vi "Initialize 8 NEO Swerve Drive.vi"() -> (0 "error out":errorcluster, 3 "Motors":T1={"Drive Motors (NEO)"={"Left Front"={"DeviceStatus"={"status"=FALSE, "code"=0, "source"=""}, "Type"=enum."PWM", "PWM"={"PWM Channel"=enum."Invalid", "DeadBand"={"Name"="", "maxPositivePwm"=0, "minPositivePwm"=0, "centerPwm"=0, "maxNegativePwm"=0, "minNegativePwm"=0, "angularRange"=0}}, "CAN"={"Device Number"=0, "SetOutput VI Ref"=variant, "GetOutput VI Ref"=variant, "Enable VI Ref"=variant, "Disable VI Ref"=variant, "Data"=variant}, "Invert"=FALSE, "DIO PWM"={"PWM \"Enable\" Channel"=enum."Invalid", "DIOChannel"=enum."Invalid", "PWM Rate"=0.0}}, "Left Back"={"DeviceStatus"={"status"=FALSE, "code"=0, "source"=""}, "Type"=enum."PWM", "PWM"={"PWM Channel"=enum."Invalid", "DeadBand"={"Name"="", "maxPositivePwm"=0, "minPositivePwm"=0, "centerPwm"=0, "maxNegativePwm"=0, "minNegativePwm"=0, "angularRange"=0}}, "CAN"={"Device Number"=0, "SetOutput VI Ref"=variant, "GetOutput VI Ref"=variant, "Enable VI Ref"=variant, "Disable VI Ref"=variant, "Data"=variant}, "Invert"=FALSE, "DIO PWM"={"PWM \"Enable\" Channel"=enum."Invalid", "DIOChannel"=enum."Invalid", "PWM Rate"=0.0}}, "Right Front"={"DeviceStatus"={"status"=FALSE, "code"=0, "source"=""}, "Type"=enum."PWM", "PWM"={"PWM Channel"=enum."Invalid", "DeadBand"={"Name"="", "maxPositivePwm"=0, "minPositivePwm"=0, "centerPwm"=0, "maxNegativePwm"=0, "minNegativePwm"=0, "angularRange"=0}}, "CAN"={"Device Number"=0, "SetOutput VI Ref"=variant, "GetOutput VI Ref"=variant, "Enable VI Ref"=variant, "Disable VI Ref"=variant, "Data"=variant}, "Invert"=FALSE, "DIO PWM"={"PWM \"Enable\" Channel"=enum."Invalid", "DIOChannel"=enum."Invalid", "PWM Rate"=0.0}}, "Right Back"={"DeviceStatus"={"status"=FALSE, "code"=0, "source"=""}, "Type"=enum."PWM", "PWM"={"PWM Channel"=enum."Invalid", "DeadBand"={"Name"="", "maxPositivePwm"=0, "minPositivePwm"=0, "centerPwm"=0, "maxNegativePwm"=0, "minNegativePwm"=0, "angularRange"=0}}, "CAN"={"Device Number"=0, "SetOutput VI Ref"=variant, "GetOutput VI Ref"=variant, "Enable VI Ref"=variant, "Disable VI Ref"=variant, "Data"=variant}, "Invert"=FALSE, "DIO PWM"={"PWM \"Enable\" Channel"=enum."Invalid", "DIOChannel"=enum."Invalid", "PWM Rate"=0.0}}}, "Steer Motors (NEO)"={"Left Front"={"DeviceStatus"={"status"=FALSE, "code"=0, "source"=""}, "Type"=enum."PWM", "PWM"={"PWM Channel"=enum."Invalid", "DeadBand"={"Name"="", "maxPositivePwm"=0, "minPositivePwm"=0, "centerPwm"=0, "maxNegativePwm"=0, "minNegativePwm"=0, "angularRange"=0}}, "CAN"={"Device Number"=0, "SetOutput VI Ref"=variant, "GetOutput VI Ref"=variant, "Enable VI Ref"=variant, "Disable VI Ref"=variant, "Data"=variant}, "Invert"=FALSE, "DIO PWM"={"PWM \"Enable\" Channel"=enum."Invalid", "DIOChannel"=enum."Invalid", "PWM Rate"=0.0}}, "Left Back"={"DeviceStatus"={"status"=FALSE, "code"=0, "source"=""}, "Type"=enum."PWM", "PWM"={"PWM Channel"=enum."Invalid", "DeadBand"={"Name"="", "maxPositivePwm"=0, "minPositivePwm"=0, "centerPwm"=0, "maxNegativePwm"=0, "minNegativePwm"=0, "angularRange"=0}}, "CAN"={"Device Number"=0, "SetOutput VI Ref"=variant, "GetOutput VI Ref"=variant, "Enable VI Ref"=variant, "Disable VI Ref"=variant, "Data"=variant}, "Invert"=FALSE, "DIO PWM"={"PWM \"Enable\" Channel"=enum."Invalid", "DIOChannel"=enum."Invalid", "PWM Rate"=0.0}}, "Right Front"={"DeviceStatus"={"status"=FALSE, "code"=0, "source"=""}, "Type"=enum."PWM", "PWM"={"PWM Channel"=enum."Invalid", "DeadBand"={"Name"="", "maxPositivePwm"=0, "minPositivePwm"=0, "centerPwm"=0, "maxNegativePwm"=0, "minNegativePwm"=0, "angularRange"=0}}, "CAN"={"Device Number"=0, "SetOutput VI Ref"=variant, "GetOutput VI Ref"=variant, "Enable VI Ref"=variant, "Disable VI Ref"=variant, "Data"=variant}, "Invert"=FALSE, "DIO PWM"={"PWM \"Enable\" Channel"=enum."Invalid", "DIOChannel"=enum."Invalid", "PWM Rate"=0.0}}, "Right Back"={"DeviceStatus"={"status"=FALSE, "code"=0, "source"=""}, "Type"=enum."PWM", "PWM"={"PWM Channel"=enum."Invalid", "DeadBand"={"Name"="", "maxPositivePwm"=0, "minPositivePwm"=0, "centerPwm"=0, "maxNegativePwm"=0, "minNegativePwm"=0, "angularRange"=0}}, "CAN"={"Device Number"=0, "SetOutput VI Ref"=variant, "GetOutput VI Ref"=variant, "Enable VI Ref"=variant, "Disable VI Ref"=variant, "Data"=variant}, "Invert"=FALSE, "DIO PWM"={"PWM \"Enable\" Channel"=enum."Invalid", "DIOChannel"=enum."Invalid", "PWM Rate"=0.0}}}, "PigeonIMUDevRef"={"DeviceStatus"={"status"=FALSE, "code"=0, "source"=""}, "Device Number"=0, "Type"=352321536, "Device ID"=0, "Handle"=0, "UsageFrame"=0, "Library Path"=path ""}, "Radii (ft)"={"Left Front Position"=[], "Left Back Position"=[], "Right Front Position"=[], "Right Back Position"=[]}} {"PigeonIMUDevRef"."Type" items=["CAN"=352321536, "TalonSRX"=33554432]; "Radii (ft)"."Right Back Position" format="%.2f"; "Radii (ft)"."Right Front Position" format="%.2f"; "Radii (ft)"."Left Back Position" format="%.2f"; "Radii (ft)"."Left Front Position" format="%.2f"})   [LabVIEW 2025]
doc: "Creates a cluster of 4 motors (order is left-front, left-back, right-front, right-back) initialized with PID coefficients and status frame reduction"
uses:
  Type Definitions/Hardware/Swerve Drives/(NEO-NEO-ThroughBore-Pigeon2) Swerve.ctl
  Type Definitions/Hardware/4 Motor Sets/(NEO & NEO 550) 4 Motor Set.ctl
  <vilib>/Rock Robotics/WPI/MotorControl/WPI_MotorControlDeviceRef.ctl
  <vilib>/Rock Robotics/WPI/MotorControl/WPI_MotorControlType.ctl
  <vilib>/Rock Robotics/SystemInterfaces/DIO/FPGA_DIOPWMChannel.ctl
  <vilib>/Rock Robotics/WPI/PWM/WPI_PWMDeadband.ctl
  <vilib>/Rock Robotics/SystemInterfaces/DIO/FPGA_DIOChannel.ctl
  <vilib>/Rock Robotics/WPI/ThirdParty/Phoenix-LabVIEW/Pigeon IMU/CTRE_PigeonIMU_DeviceRef.ctl
  <vilib>/Rock Robotics/WPI/ThirdParty/Phoenix-LabVIEW/Pigeon IMU/CTRE_PigeonIMU_ConnectionType.ctl
  Type Definitions/Data/Pod Positions.ctl
  Type Definitions/Hardware/Swerve Configs/NEO-NEO-ThroughBore-Pigeon2 Swerve Config.ctl
  <vilib>/Rock Robotics/WPI/ThirdParty/REV Robotics/REVLib/Typedef/SPARK Feed Forward Gains.ctl
  <vilib>/Rock Robotics/WPI/ThirdParty/REV Robotics/REVLib/Typedef/Spark MAX Idle Mode.ctl
  <vilib>/Rock Robotics/WPI/ThirdParty/REV Robotics/REVLib/Typedef/SPARK Feedback Sensor.ctl
  <vilib>/Rock Robotics/WPI/ThirdParty/REV Robotics/REVLib/Typedef/Spark MAX Status Frames.ctl
  <vilib>/Rock Robotics/WPI/ThirdParty/REV Robotics/REVLib/Typedef/Closed Loop Voltage Mode.ctl
  <vilib>/Rock Robotics/WPI/ThirdParty/REV Robotics/REVLib/Typedef/Spark MAX Hall Sensor Average Depth Size.ctl
  <vilib>/Rock Robotics/WPI/ThirdParty/REV Robotics/REVLib/SubVI/Public/SPARK Open Brushless.vi
  <vilib>/Rock Robotics/WPI/ThirdParty/REV Robotics/REVLib/SubVI/Public/SPARK Configure Power Smart Current Limit.vi
  <vilib>/Rock Robotics/WPI/ThirdParty/REV Robotics/REVLib/SubVI/Public/SPARK Configure Closed Loop Basic.vi
  <vilib>/Rock Robotics/WPI/ThirdParty/REV Robotics/REVLib/SubVI/Public/SPARK Configure Encoder Conversion Factors.vi
  <vilib>/Rock Robotics/WPI/ThirdParty/REV Robotics/REVLib/SubVI/Public/SPARK Configure Closed Loop Position Wrapping.vi
  <vilib>/Rock Robotics/WPI/ThirdParty/REV Robotics/REVLib/SubVI/Public/SPARK Configure Basic Idle Mode.vi
  <vilib>/Rock Robotics/WPI/ThirdParty/REV Robotics/REVLib/SubVI/Public/SPARK Configure Closed Loop Voltage Mode.vi
  <vilib>/Rock Robotics/WPI/ThirdParty/REV Robotics/REVLib/SubVI/Public/SPARK Configure Encoder Velocity Filtering UVW.vi
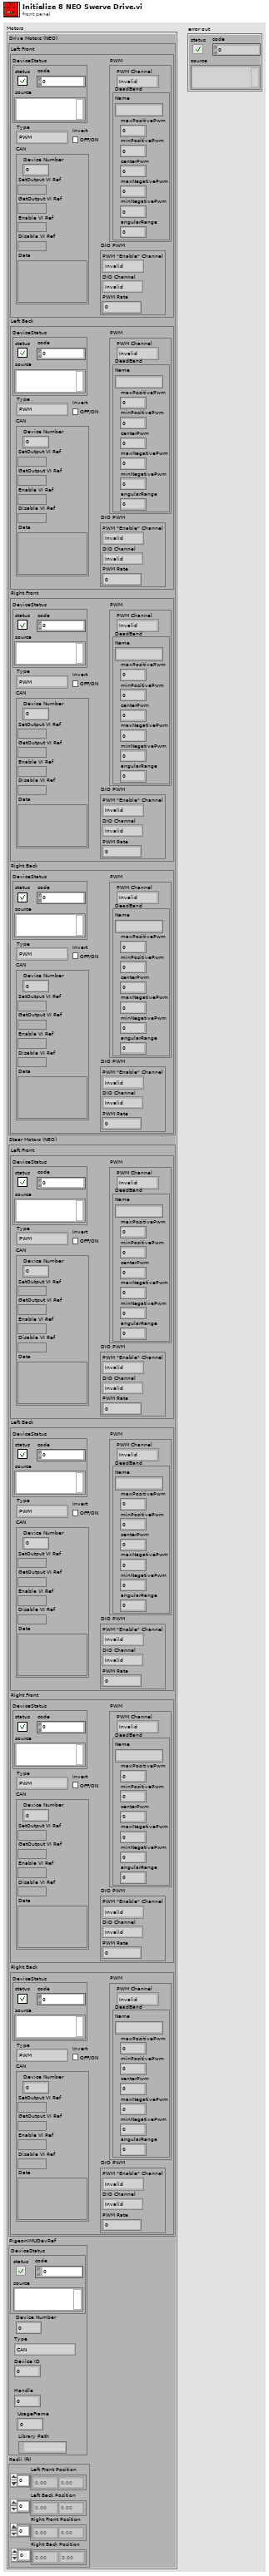
[diagram p1: front panel]
types:
  T1 = typedef "(NEO-NEO-ThroughBore-Pigeon2) Swerve.ctl" = cluster{"Drive Motors (NEO)":T2, "Steer Motors (NEO)":T2, "PigeonIMUDevRef":T8, "Radii (ft)":T10}
  T2 = typedef "(NEO & NEO 550) 4 Motor Set.ctl" = cluster{"Left Front":T3, "Left Back":T3, "Right Front":T3, "Right Back":T3}
  T3 = typedef "WPI_MotorControlDeviceRef.ctl" = cluster{"DeviceStatus":errorcluster, "Type":T4, "PWM":cluster{"PWM Channel":T5, "DeadBand":T6}, "CAN":cluster{"Device Number":u8, "SetOutput VI Ref":variant, "GetOutput VI Ref":variant, "Enable VI Ref":variant, "Disable VI Ref":variant, "Data":variant}, "Invert":bool, "DIO PWM":cluster{"PWM \"Enable\" Channel":T5, "DIOChannel":T7, "PWM Rate":dbl}}
  T4 = typedef "WPI_MotorControlType.ctl" = enum16{"PWM", "CAN", "DIO PWM"}
  T5 = typedef "FPGA_DIOPWMChannel.ctl" = enum8{"PWM 0", "PWM 1", "PWM 2", "PWM 3", "PWM 4", "PWM 5", "PWM 6", "PWM 7", "PWM 8", "PWM 9", "PWM MXP 0", "PWM MXP 1", "PWM MXP 2", "PWM MXP 3", "PWM MXP 4", "PWM MXP 5", "PWM MXP 6", "PWM MXP 7", "PWM MXP 8", "PWM MXP 9", "Invalid"}
  T6 = typedef "WPI_PWMDeadband.ctl" = cluster{"Name":string, "maxPositivePwm":i32, "minPositivePwm":i32, "centerPwm":i32, "maxNegativePwm":i32, "minNegativePwm":i32, "angularRange":u16}
  T7 = typedef "FPGA_DIOChannel.ctl" = enum8{"DIO 0", "DIO 1", "DIO 2", "DIO 3", "DIO 4", "DIO 5", "DIO 6", "DIO 7", "DIO 8", "DIO 9", "DIO MXP 0", "DIO MXP 1", "DIO MXP 2", "DIO MXP 3", "DIO MXP 4", "DIO MXP 5", "DIO MXP 6", "DIO MXP 7", "DIO MXP 8", "DIO MXP 9", "DIO MXP 10", "DIO MXP 11", "DIO MXP 12", "DIO MXP 13", "DIO MXP 14", "DIO MXP 15", "SPI Port CS1", "SPI Port CS2", "SPI Port CS3", "SPI Port MISO", "SPI Port MOSI", "Invalid"}
  T8 = typedef "CTRE_PigeonIMU_DeviceRef.ctl" = cluster{"DeviceStatus":errorcluster, "Device Number":u8, "Type":T9, "Device ID":u32, "Handle":u64, "UsageFrame":u32, "Library Path":path}
  T9 = typedef "CTRE_PigeonIMU_ConnectionType.ctl" = u32
  T10 = typedef "Pod Positions.ctl" = cluster{"Left Front Position":dbl[], "Left Back Position":dbl[], "Right Front Position":dbl[], "Right Back Position":dbl[]}
  T11 = typedef "NEO-NEO-ThroughBore-Pigeon2 Swerve Config.ctl" = cluster{"Drive Motor CAN IDs":cluster{"LF CAN ID":dbl, "LB CAN ID":dbl, "RF CAN ID":dbl, "RB CAN ID":dbl}, "Steer Motor CAN IDs":cluster{"LF CAN ID":dbl, "LB CAN ID":dbl, "RF CAN ID":dbl, "RB CAN ID":dbl}, "Drive PID Gains":cluster{cluster{"P Gain":dbl, "I Gain":dbl, "D Gain":dbl}, "Feed Forward Gains":T12, "I Zone":dbl, "Min Output":dbl, "Max Output":dbl}, "Steer PID Gains":cluster{cluster{"P Gain":dbl, "I Gain":dbl, "D Gain":dbl}, "Feed Forward Gains":T12, "I Zone":dbl, "Min Output":dbl, "Max Output":dbl}, "Pigeon 2 Refnum":string, "Pod Locations (ft)":T10}
  T12 = typedef "SPARK Feed Forward Gains.ctl" = cluster{"kV":dbl, "kS":dbl, "kA":dbl, "kG":dbl, "kCos":dbl, "kCosRatio":dbl}
  T13 = cluster{"LF CAN ID":dbl, "LB CAN ID":dbl, "RF CAN ID":dbl, "RB CAN ID":dbl}
  T14 = cluster{cluster{"P Gain":dbl, "I Gain":dbl, "D Gain":dbl}, "Feed Forward Gains":T12, "I Zone":dbl, "Min Output":dbl, "Max Output":dbl}
  T15 = typedef "Spark MAX Hall Sensor Average Depth Size.ctl" = enum16{"1", "2", "4", "8"}
  T16 = typedef "SPARK Feedback Sensor.ctl" = enum16{"No Sensor", "Primary Encoder", "Analog Sensor", "Alternate or External Encoder", "Duty Cycle Sensor"}
  T17 = typedef "Closed Loop Voltage Mode.ctl" = enum16{"Disabled", "Voltage Output", "Voltage Compensation"}
  T18 = typedef "Spark MAX Status Frames.ctl" = enum16{"Status 0", "Status 1", "Status 2", "Status 3", "Status 4", "Status 5", "Status 6", "Status 7"}
  T19 = typedef "Spark MAX Idle Mode.ctl" = enum16{"Coast", "Brake"}
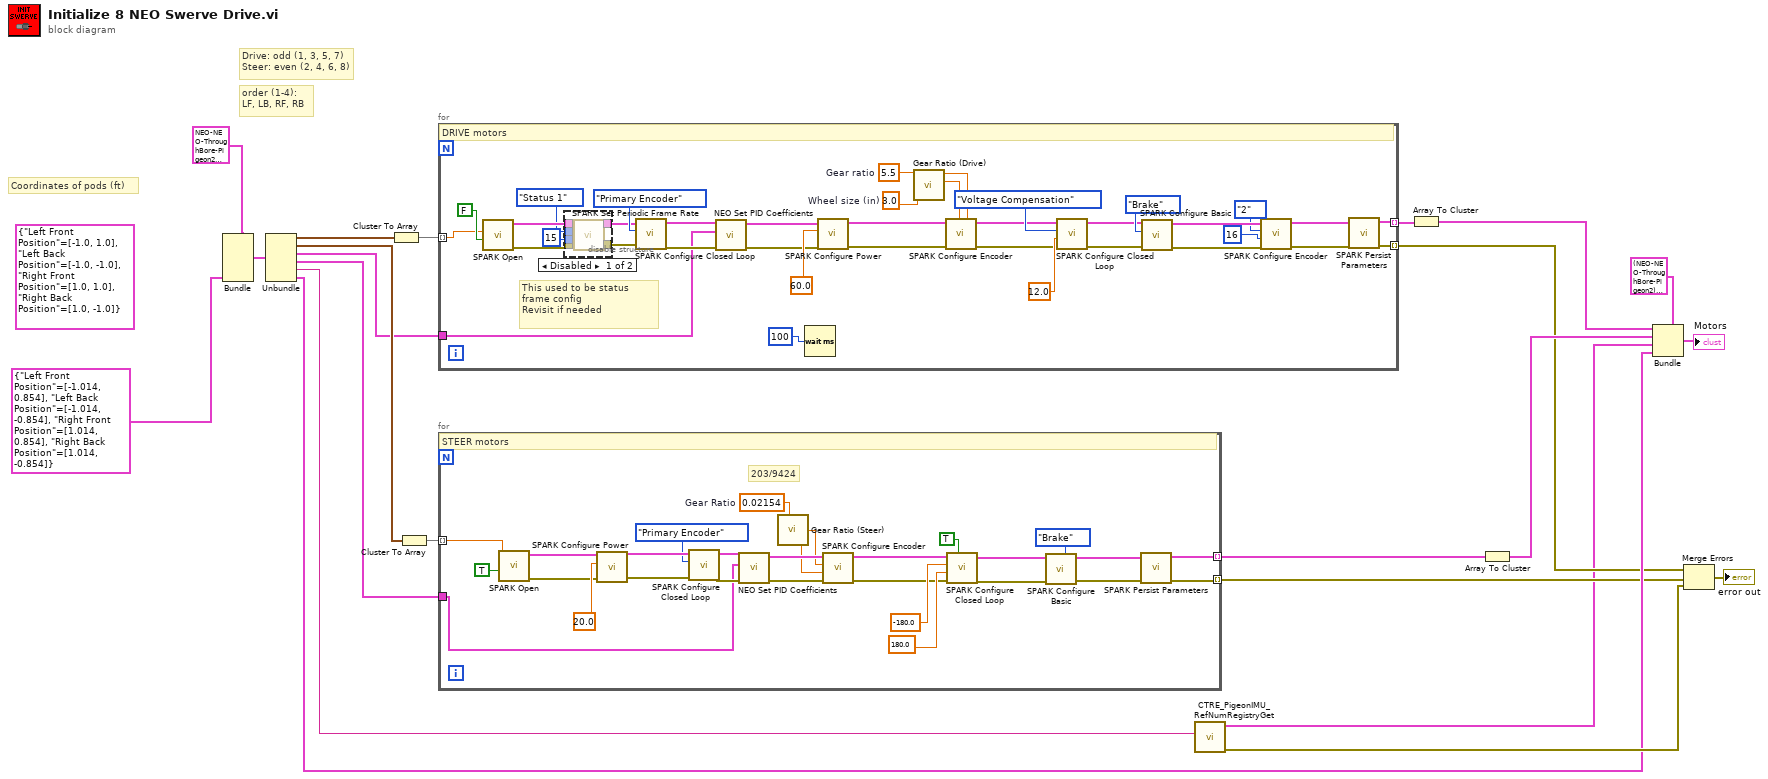
[diagram p0: block diagram]
diagram:
  (unwired) T10 {"Left Front Position"=[-1.0, 1.0], "Left Back Position"=[-1.0, -1.0], "Right Front Position"=[1.0, 1.0], "Right Back Position"=[1.0, -1.0]} ("Radii (ft)")
  # "Drive: odd (1, 3, 5, 7)\nSteer: even (2, 4, 6, 8)"
  # "Coordinates of pods (ft)"
  # "order (1-4):\nLF, LB, RF, RB"
  n1 = Bundle(cluster=T11 {"Drive Motor CAN IDs"={"LF CAN ID"=1.0, "LB CAN ID"=3.0, "RF CAN ID"=5.0, "RB CAN ID"=7.0}, "Steer Motor CAN IDs"={"LF CAN ID"=2.0, "LB CAN ID"=4.0, "RF CAN ID"=6.0, "RB CAN ID"=8.0}, "Drive PID Gains"={{"P Gain"=0.12, "I Gain"=0.0, "D Gain"=0.0}, "Feed Forward Gains"={"kV"=0.08, "kS"=0.0, "kA"=0.0, "kG"=0.0, "kCos"=0.0, "kCosRatio"=0.0}, "I Zone"=0.0, "Min Output"=-1.0, "Max Output"=1.0}, "Steer PID Gains"={{"P Gain"=0.08, "I Gain"=0.0, "D Gain"=0.0}, "Feed Forward Gains"={"kV"=0.0, "kS"=0.0, "kA"=0.0, "kG"=0.0, "kCos"=0.0, "kCosRatio"=0.0}, "I Zone"=0.0, "Min Output"=-1.0, "Max Output"=1.0}, "Pigeon 2 Refnum"="IMU", "Pod Locations (ft)"={"Left Front Position"=[], "Left Back Position"=[], "Right Front Position"=[], "Right Back Position"=[]}} ("Swerve Config"), "Pod Locations (ft)"=T10 {"Left Front Position"=[-1.014, 0.854], "Left Back Position"=[-1.014, -0.854], "Right Front Position"=[1.014, 0.854], "Right Back Position"=[1.014, -0.854]} ("Radii (ft)")) -> (w18:T11)  [unwired: 5 in]
  n2 = Unbundle(w18) -> ("Drive Motor CAN IDs"=w17:T13, "Steer Motor CAN IDs"=w16:T13, "Drive PID Gains"=w13:T14, "Steer PID Gains"=w12:T14, "Pigeon 2 Refnum"=w11:string, "Pod Locations (ft)"=w10:T10)
  n3 = Cluster To Array(cluster=w17) -> (array=w22:dbl[])
  n4 = Cluster To Array(cluster=w16) -> (array=w21:dbl[])
  n5 = for {
    tunnel: w22 -> [w33] mode=indexing
    tunnel: w13 -> [w27]
    tunnel: [w24] -> w8 mode=indexing
    tunnel: [w23] -> w4 mode=indexing
    w53 = 3.0  # Wheel size (in)
    w56 = 5.5  # Gear ratio
    # "This used to be status frame config\nRevisit if needed"
    # "DRIVE motors"
    n6 = call-poly <vilib>:"SPARK Open.vi"("Invert"=FALSE, "Device Number"=w33) -> ("error out"=w57:errorcluster, "MotorControlDeviceRef"=w58:T3)  [unwired: 8 in]
    n7 = disable-structure shown="Disabled" {
      disable-tunnel: w58 -> [w63 w65]
      disable-tunnel: w57 -> [w62 w64]
      disable-tunnel: u16 15 ("Frame rate (ms)") -> [w61 _]
      disable-tunnel: Spark_MAX_Status_Frames."Status 1" ("Frame") -> [w60 _]
      disable-tunnel: [_ w65] -> w37
      disable-tunnel: [_ w64] -> w36
      frame Disabled {
        n8 = call <vilib>:"SPARK Set Periodic Frame Rate.vi"("error in"=w62, "Frame rate (ms)"=w61, "Frame"=w60, "MotorControlDeviceRef"=w63) -> ()  [unwired: 6 in, 2 out]
      }
      frame Enabled {
      }
    }
    n9 = call-poly <vilib>:"SPARK Configure Closed Loop.vi"("error in"=w36, "Feedback Sensor (Primary Encoder)"=SPARK_Feedback_Sensor."Primary Encoder", "MotorControlDeviceRef in"=w37) -> ("error out"=w29:errorcluster, "MotorControlDeviceRef out"=w32:T3)  [unwired: 7 in]
    n10 = call "NEO Set PID Coefficients.vi"("error in"=w29, "PID Gains"=w27, "MotorControlDeviceRef in"=w32) -> ("error out"=w30:errorcluster, "MotorControlDeviceRef out"=w31:T3)  [unwired: 5 in]
    n11 = Wait (ms)(milliseconds to wait=u32 100) -> ()  [unwired: 1 out]
    n12 = call-poly <vilib>:"SPARK Configure Power.vi"("error in (no error)"=w30, "Primay Current Limit (80A)"=60.0, "MotorControlDeviceRef in"=w31) -> ("error out"=w41:errorcluster, "MotorControlDeviceRef out"=w42:T3)  [unwired: 7 in]
    n13 = call "Gear Ratio (Drive).vi"("Wheel size (in)"=w53, "Gear ratio"=w56) -> ("Position Factor"=w54:dbl, "Velocity Factor (ft/s)"=w55:dbl)  [unwired: 8 in]
    n14 = call-poly <vilib>:"SPARK Configure Encoder.vi"("error in"=w41, "Velocity Conversion Factor"=w55, "Position Conversion Factor"=w54, "MotorControlDeviceRef in"=w42) -> ("error out"=w43:errorcluster, "MotorControlDeviceRef out"=w44:T3)  [unwired: 6 in]
    n15 = call-poly <vilib>:"SPARK Configure Closed Loop.vi"("error in (no error)"=w43, "Compensated Nominal Voltage"=12.0 ("Nominal Voltage"), "Voltage Mode (Disabled)"=Closed_Loop_Voltage_Mode."Voltage Compensation", "MotorControlDeviceRef in"=w44) -> ("error out"=w45:errorcluster, "MotorControlDeviceRef out"=w46:T3)  [unwired: 6 in]
    n16 = call-poly <vilib>:"SPARK Configure Basic.vi"("error in (no error)"=w45, "Idle Mode"=Spark_MAX_Idle_Mode."Brake", "MotorControlDeviceRef in"=w46) -> ("error out"=w39:errorcluster, "MotorControlDeviceRef out"=w40:T3)  [unwired: 7 in]
    n17 = call-poly <vilib>:"SPARK Configure Encoder.vi"("error in"=w39, "Measurement Period (ms)"=u32 16, "Average Depth (8)"=Spark_MAX_Hall_Sensor_Average_Depth_Size."2", "MotorControlDeviceRef in"=w40) -> ("error out"=w25:errorcluster, "MotorControlDeviceRef out"=w26:T3)  [unwired: 6 in]
    n18 = call <vilib>:"SPARK Persist Parameters.vi"("error in"=w25, "MotorControlDeviceRef"=w26) -> ("error out"=w23:errorcluster, "MotorControlDeviceRef"=w24:T3)  [unwired: 8 in]
  }
  n19 = for {
    tunnel: w21 -> [w93] mode=indexing
    tunnel: w12 -> [w73]
    tunnel: [w68] -> w6 mode=indexing
    tunnel: [w66] -> w5 mode=indexing
    w70 = 0.02154  # Gear Ratio
    # "203/9424"
    # "STEER motors"
    n20 = call-poly <vilib>:"SPARK Open.vi"("Invert"=TRUE, "Device Number"=w93) -> ("error out"=w81:errorcluster, "MotorControlDeviceRef"=w82:T3)  [unwired: 8 in]
    n21 = call-poly <vilib>:"SPARK Configure Power.vi"("error in (no error)"=w81, "Primay Current Limit (80A)"=20.0, "MotorControlDeviceRef in"=w82) -> ("error out"=w75:errorcluster, "MotorControlDeviceRef out"=w76:T3)  [unwired: 7 in]
    n22 = call-poly <vilib>:"SPARK Configure Closed Loop.vi"("error in"=w75, "Feedback Sensor (Primary Encoder)"=SPARK_Feedback_Sensor."Primary Encoder", "MotorControlDeviceRef in"=w76) -> ("error out"=w77:errorcluster, "MotorControlDeviceRef out"=w80:T3)  [unwired: 7 in]
    n23 = call "NEO Set PID Coefficients.vi"("error in"=w77, "PID Gains"=w73, "MotorControlDeviceRef in"=w80) -> ("error out"=w78:errorcluster, "MotorControlDeviceRef out"=w79:T3)  [unwired: 5 in]
    n24 = call "Gear Ratio (Steer).vi"("Gear Ratio"=w70) -> ("Position Factor"=w72:dbl, "Velocity Factor"=w71:dbl)  [unwired: 6 in]
    n25 = call-poly <vilib>:"SPARK Configure Encoder.vi"("error in"=w78, "Velocity Conversion Factor"=w71, "Position Conversion Factor"=w72, "MotorControlDeviceRef in"=w79) -> ("error out"=w83:errorcluster, "MotorControlDeviceRef out"=w84:T3)  [unwired: 6 in]
    n26 = call-poly <vilib>:"SPARK Configure Closed Loop.vi"("Enable (T)"=TRUE ("Enable (F)"), "error in"=w83, "Maximum Input"=180.0 ("Maximum Output (0)"), "Minimum Input"=-180.0 ("Minimum Input (0)"), "MotorControlDeviceRef in"=w84) -> ("error out"=w85:errorcluster, "MotorControlDeviceRef out"=w86:T3)  [unwired: 5 in]
    n27 = call-poly <vilib>:"SPARK Configure Basic.vi"("error in (no error)"=w85, "Idle Mode"=Spark_MAX_Idle_Mode."Brake", "MotorControlDeviceRef in"=w86) -> ("error out"=w67:errorcluster, "MotorControlDeviceRef out"=w69:T3)  [unwired: 7 in]
    n28 = call <vilib>:"SPARK Persist Parameters.vi"("error in"=w67, "MotorControlDeviceRef"=w69) -> ("error out"=w66:errorcluster, "MotorControlDeviceRef"=w68:T3)  [unwired: 8 in]
  }
  n29 = call <vilib>:"CTRE_PigeonIMU_RefNumRegistryGet.vi"("refnum name"=w11) -> ("error out"=w15:errorcluster, "PigeonIMUDevRef"=w1:T8)  [unwired: 9 in]
  n30 = Array To Cluster(array=w8) -> (cluster=w3:cluster{"[0]":T3, "[1]":T3, "[2]":T3, "[3]":T3})
  n31 = Array To Cluster(array=w6) -> (cluster=w7:cluster{"[0]":T3, "[1]":T3, "[2]":T3, "[3]":T3})
  n32 = Bundle(cluster=T1 {"Drive Motors (NEO)"={"Left Front"={"DeviceStatus"={"status"=FALSE, "code"=0, "source"=""}, "Type"=enum."PWM", "PWM"={"PWM Channel"=enum."Invalid", "DeadBand"={"Name"="", "maxPositivePwm"=0, "minPositivePwm"=0, "centerPwm"=0, "maxNegativePwm"=0, "minNegativePwm"=0, "angularRange"=0}}, "CAN"={"Device Number"=0, "SetOutput VI Ref"=variant, "GetOutput VI Ref"=variant, "Enable VI Ref"=variant, "Disable VI Ref"=variant, "Data"=variant}, "Invert"=FALSE, "DIO PWM"={"PWM \"Enable\" Channel"=enum."Invalid", "DIOChannel"=enum."Invalid", "PWM Rate"=0.0}}, "Left Back"={"DeviceStatus"={"status"=FALSE, "code"=0, "source"=""}, "Type"=enum."PWM", "PWM"={"PWM Channel"=enum."Invalid", "DeadBand"={"Name"="", "maxPositivePwm"=0, "minPositivePwm"=0, "centerPwm"=0, "maxNegativePwm"=0, "minNegativePwm"=0, "angularRange"=0}}, "CAN"={"Device Number"=0, "SetOutput VI Ref"=variant, "GetOutput VI Ref"=variant, "Enable VI Ref"=variant, "Disable VI Ref"=variant, "Data"=variant}, "Invert"=FALSE, "DIO PWM"={"PWM \"Enable\" Channel"=enum."Invalid", "DIOChannel"=enum."Invalid", "PWM Rate"=0.0}}, "Right Front"={"DeviceStatus"={"status"=FALSE, "code"=0, "source"=""}, "Type"=enum."PWM", "PWM"={"PWM Channel"=enum."Invalid", "DeadBand"={"Name"="", "maxPositivePwm"=0, "minPositivePwm"=0, "centerPwm"=0, "maxNegativePwm"=0, "minNegativePwm"=0, "angularRange"=0}}, "CAN"={"Device Number"=0, "SetOutput VI Ref"=variant, "GetOutput VI Ref"=variant, "Enable VI Ref"=variant, "Disable VI Ref"=variant, "Data"=variant}, "Invert"=FALSE, "DIO PWM"={"PWM \"Enable\" Channel"=enum."Invalid", "DIOChannel"=enum."Invalid", "PWM Rate"=0.0}}, "Right Back"={"DeviceStatus"={"status"=FALSE, "code"=0, "source"=""}, "Type"=enum."PWM", "PWM"={"PWM Channel"=enum."Invalid", "DeadBand"={"Name"="", "maxPositivePwm"=0, "minPositivePwm"=0, "centerPwm"=0, "maxNegativePwm"=0, "minNegativePwm"=0, "angularRange"=0}}, "CAN"={"Device Number"=0, "SetOutput VI Ref"=variant, "GetOutput VI Ref"=variant, "Enable VI Ref"=variant, "Disable VI Ref"=variant, "Data"=variant}, "Invert"=FALSE, "DIO PWM"={"PWM \"Enable\" Channel"=enum."Invalid", "DIOChannel"=enum."Invalid", "PWM Rate"=0.0}}}, "Steer Motors (NEO)"={"Left Front"={"DeviceStatus"={"status"=FALSE, "code"=0, "source"=""}, "Type"=enum."PWM", "PWM"={"PWM Channel"=enum."Invalid", "DeadBand"={"Name"="", "maxPositivePwm"=0, "minPositivePwm"=0, "centerPwm"=0, "maxNegativePwm"=0, "minNegativePwm"=0, "angularRange"=0}}, "CAN"={"Device Number"=0, "SetOutput VI Ref"=variant, "GetOutput VI Ref"=variant, "Enable VI Ref"=variant, "Disable VI Ref"=variant, "Data"=variant}, "Invert"=FALSE, "DIO PWM"={"PWM \"Enable\" Channel"=enum."Invalid", "DIOChannel"=enum."Invalid", "PWM Rate"=0.0}}, "Left Back"={"DeviceStatus"={"status"=FALSE, "code"=0, "source"=""}, "Type"=enum."PWM", "PWM"={"PWM Channel"=enum."Invalid", "DeadBand"={"Name"="", "maxPositivePwm"=0, "minPositivePwm"=0, "centerPwm"=0, "maxNegativePwm"=0, "minNegativePwm"=0, "angularRange"=0}}, "CAN"={"Device Number"=0, "SetOutput VI Ref"=variant, "GetOutput VI Ref"=variant, "Enable VI Ref"=variant, "Disable VI Ref"=variant, "Data"=variant}, "Invert"=FALSE, "DIO PWM"={"PWM \"Enable\" Channel"=enum."Invalid", "DIOChannel"=enum."Invalid", "PWM Rate"=0.0}}, "Right Front"={"DeviceStatus"={"status"=FALSE, "code"=0, "source"=""}, "Type"=enum."PWM", "PWM"={"PWM Channel"=enum."Invalid", "DeadBand"={"Name"="", "maxPositivePwm"=0, "minPositivePwm"=0, "centerPwm"=0, "maxNegativePwm"=0, "minNegativePwm"=0, "angularRange"=0}}, "CAN"={"Device Number"=0, "SetOutput VI Ref"=variant, "GetOutput VI Ref"=variant, "Enable VI Ref"=variant, "Disable VI Ref"=variant, "Data"=variant}, "Invert"=FALSE, "DIO PWM"={"PWM \"Enable\" Channel"=enum."Invalid", "DIOChannel"=enum."Invalid", "PWM Rate"=0.0}}, "Right Back"={"DeviceStatus"={"status"=FALSE, "code"=0, "source"=""}, "Type"=enum."PWM", "PWM"={"PWM Channel"=enum."Invalid", "DeadBand"={"Name"="", "maxPositivePwm"=0, "minPositivePwm"=0, "centerPwm"=0, "maxNegativePwm"=0, "minNegativePwm"=0, "angularRange"=0}}, "CAN"={"Device Number"=0, "SetOutput VI Ref"=variant, "GetOutput VI Ref"=variant, "Enable VI Ref"=variant, "Disable VI Ref"=variant, "Data"=variant}, "Invert"=FALSE, "DIO PWM"={"PWM \"Enable\" Channel"=enum."Invalid", "DIOChannel"=enum."Invalid", "PWM Rate"=0.0}}}, "PigeonIMUDevRef"={"DeviceStatus"={"status"=FALSE, "code"=0, "source"=""}, "Device Number"=0, "Type"=352321536, "Device ID"=0, "Handle"=0, "UsageFrame"=0, "Library Path"=path ""}, "Radii (ft)"={"Left Front Position"=[], "Left Back Position"=[], "Right Front Position"=[], "Right Back Position"=[]}} ("(N-N-C-P) Swerve Motors"), "Drive Motors (NEO)"=w3, "Steer Motors (NEO)"=w7, "PigeonIMUDevRef"=w1, "Radii (ft)"=w10) -> (→"Motors":T1)
  n33 = Merge Errors(w4, w5, w15) -> (→"error out":errorcluster)
